vi "Simulate_AirGaps_v1_Core.vi"() -> ()   [LabVIEW 2014]
doc: "I. Description:\nThis example demonstrates how to continuously output a waveform using an internal sample clock. The automatic regeneration of data has been disabled, so new data has to be provided throughout the duration of the continuous Analog Output operation. This allows the generation of any arbitrary frequency as this VI computes new data for each iteration of the loop, maintaining phase continuity of the signal.\n\nII. Instructions for Running:\n1. Select the Physical Channel to correspond to where your signal is output on the DAQ device.\n2. Enter the Minimum and Maximum Voltage range.\n3. Specify the desired Sample Clock Rate of the output Waveform. Higher sample clock rates will produce a smoother waveform.\n4. Manually specify the Analog Output buffer size, in number of samples. A larger buffer would help non-regenerative operations avoid errors due to occasional high CPU load. \nNote: \nThe Analog Output buffer has to be at least as big as the amount of data being written to the board per iteration. The recommended buffer size would be at least twice the amount of data being written to the board per iteration.\n5. Enter the Waveform Information. See the documentation of the Basic Function Generator SubVI for information on each parameter.\n\nIII. Block Diagram Steps:\n1. Create an Analog Output Voltage channel.\n2. Configure the task to prohibit the automatic regeneration of data.\n3. Call the DAQmx (Sample Clock) VI to set the sample clock rate. Additionally, set the sample mode to Continuous.\n4. Read the actual sample clock rate (eventually coerced depending on the hardware used). \n5. Compute the desired waveform, using the buffer size and the actual update rate. This VI keeps track of the phase of the waveform to ensure that the generated signal is continuous.\n6. Write the waveform to the output buffer. \n7a. Call the Start VI. This is only needed when the loop is executed for the first time.\n7b. Do nothing.\n8. Loop continuously until user presses the Stop button. Every iteration computes and writes a new waveform to the buffer.\n9. Call the Clear Task VI to clear the Task.\n10. Use the popup dialog box to display an error or warning if any.\n\nIV. I/O Connections Overview:\nMake sure your signal output terminal matches the Physical Channel I/O Control. For further connection information, refer to your hardware reference manual."
uses:
  <vilib>/Utility/error.llb/DialogType.ctl
  <vilib>/DAQmx/create/channels.llb/DAQmx Create Channel (AO-Voltage-Basic).vi
  <vilib>/DAQmx/configure/timing.llb/DAQmx Timing (Sample Clock).vi
  <vilib>/DAQmx/write.llb/DAQmx Write (Analog 1D Wfm NChan NSamp).vi
  <vilib>/measure/NI_MABase.lvlib
  <resource>/objmgr/daqmx.rc
panel:
  in  "Tab Control":T1(tab)=enum."Air Gap"
  out "Trigger":waveform(dbl)(graph)={"t0"=timestamp(90 s since 1904-01-01), "dt"=0.0005333333333333334, "Y"=array[1500 elements]}
  in  "Trigg. level":sgl=2.0
  in  "Regular level":sgl=10.0
  out "RV":waveform(dbl)[](graph)=[{"t0"=timestamp(90 s since 1904-01-01), "dt"=0.0005333333333333334, "Y"=array[1500 elements]}, {"t0"=timestamp(90 s since 1904-01-01), "dt"=0.0005333333333333334, "Y"=array[1500 elements]}, {"t0"=timestamp(90 s since 1904-01-01), "dt"=0.0005333333333333334, "Y"=array[1500 elements]}, {"t0"=timestamp(90 s since 1904-01-01), "dt"=0.0005333333333333334, "Y"=array[1500 elements]}]
  in  "RV000_Ph":sgl[](array[numeric])=[30.0, 60.0, 90.0]
  in  "RV000_Amp":sgl[](array[numeric])=[1.0, 1.0, 1.0]
  in  "RV000.DC":sgl=5.0
  in  "RV001.DC":sgl=5.0
  in  "RV001_Amp":sgl[](array[numeric])=[1.0, 1.0, 1.0]
  in  "RV001_Ph":sgl[](array[numeric])=[30.0, 60.0, 90.0]
  in  "RV002_Ph":sgl[](array[numeric])=[30.0, 60.0, 90.0]
  in  "RV002_Amp":sgl[](array[numeric])=[1.0, 1.0, 1.0]
  in  "RV002.DC":sgl=5.0
  in  "RV003_Ph":sgl[](array[numeric])=[30.0, 60.0, 90.0]
  in  "RV003_Amp":sgl[](array[numeric])=[1.0, 1.0, 1.0]
  in  "RV003.DC":sgl=5.0
  in  "Multiplication factor":dbl=0.5
  in  "Add Noise":bool
  in  "Change roattion":bool
  in  "First harmonic Phase":sgl=0.1
  out "AG_graph":waveform(dbl)[](graph)
  in  "Pole hight":sgl=6.0
  in  "Add linear increase":bool
  in  "Pole to highlight (from 1 to 72)":i32=166
  in  "Higlight multiplication factor":sgl=1.2
  in  "Offset":sgl=11.0
  in  "increase rate/rotation":sgl=0.5
  in  "Samples to rotate +/100":i32
  in  "First harmonic Amplitude":sgl=0.1
  in  "Add first harmonic":bool
  out "MX":waveform(dbl)(graph)
  in  "MX Amplitude":sgl=1.0
  in  "Pole to highlight (from 1 to 72) MX":i32=166
  in  "Higlight multiplication factor MX":sgl=1.2
  out "Proc1":waveform(dbl)(graph)={"t0"=timestamp(90 s since 1904-01-01), "dt"=0.0005333333333333334, "Y"=array[1500 elements]}
  in  "DC Proc Val 1":sgl=6.0
  out "Proc2":waveform(dbl)(graph)={"t0"=timestamp(90 s since 1904-01-01), "dt"=0.0005333333333333334, "Y"=array[1500 elements]}
  in  "DC Proc Val 2":sgl=6.0
  out "Loop Iteration":dbl=0.7980451583862305
  out "Waveform Graph":waveform(dbl)[](graph)=[{"t0"=timestamp(90 s since 1904-01-01), "dt"=0.0005333333333333334, "Y"=array[1500 elements]}, {"t0"=timestamp(90 s since 1904-01-01), "dt"=0.0005333333333333334, "Y"=array[1500 elements]}, {"t0"=timestamp(90 s since 1904-01-01), "dt"=0.0005333333333333334, "Y"=array[1500 elements]}, {"t0"=timestamp(90 s since 1904-01-01), "dt"=0.0005333333333333334, "Y"=array[1500 elements]}, {"t0"=timestamp(90 s since 1904-01-01), "dt"=0.0005333333333333334, "Y"=array[1500 elements]}, {"t0"=timestamp(90 s since 1904-01-01), "dt"=0.0005333333333333334, "Y"=array[1500 elements]}, {"t0"=timestamp(90 s since 1904-01-01), "dt"=0.0005333333333333334, "Y"=array[1500 elements]}, {"t0"=timestamp(90 s since 1904-01-01), "dt"=0.0005333333333333334, "Y"=array[1500 elements]}, {"t0"=timestamp(90 s since 1904-01-01), "dt"=0.0005333333333333334, "Y"=array[1500 elements]}, {"t0"=timestamp(90 s since 1904-01-01), "dt"=0.0005333333333333334, "Y"=array[1500 elements]}, {"t0"=timestamp(90 s since 1904-01-01), "dt"=0.0005333333333333334, "Y"=array[1500 elements]}] caption="Output Waveforms"
  in  "Physical Channels":tag="Dev2/ao0:11"
  in  "stop":bool
  # "Channel Parameters"
  # "s"
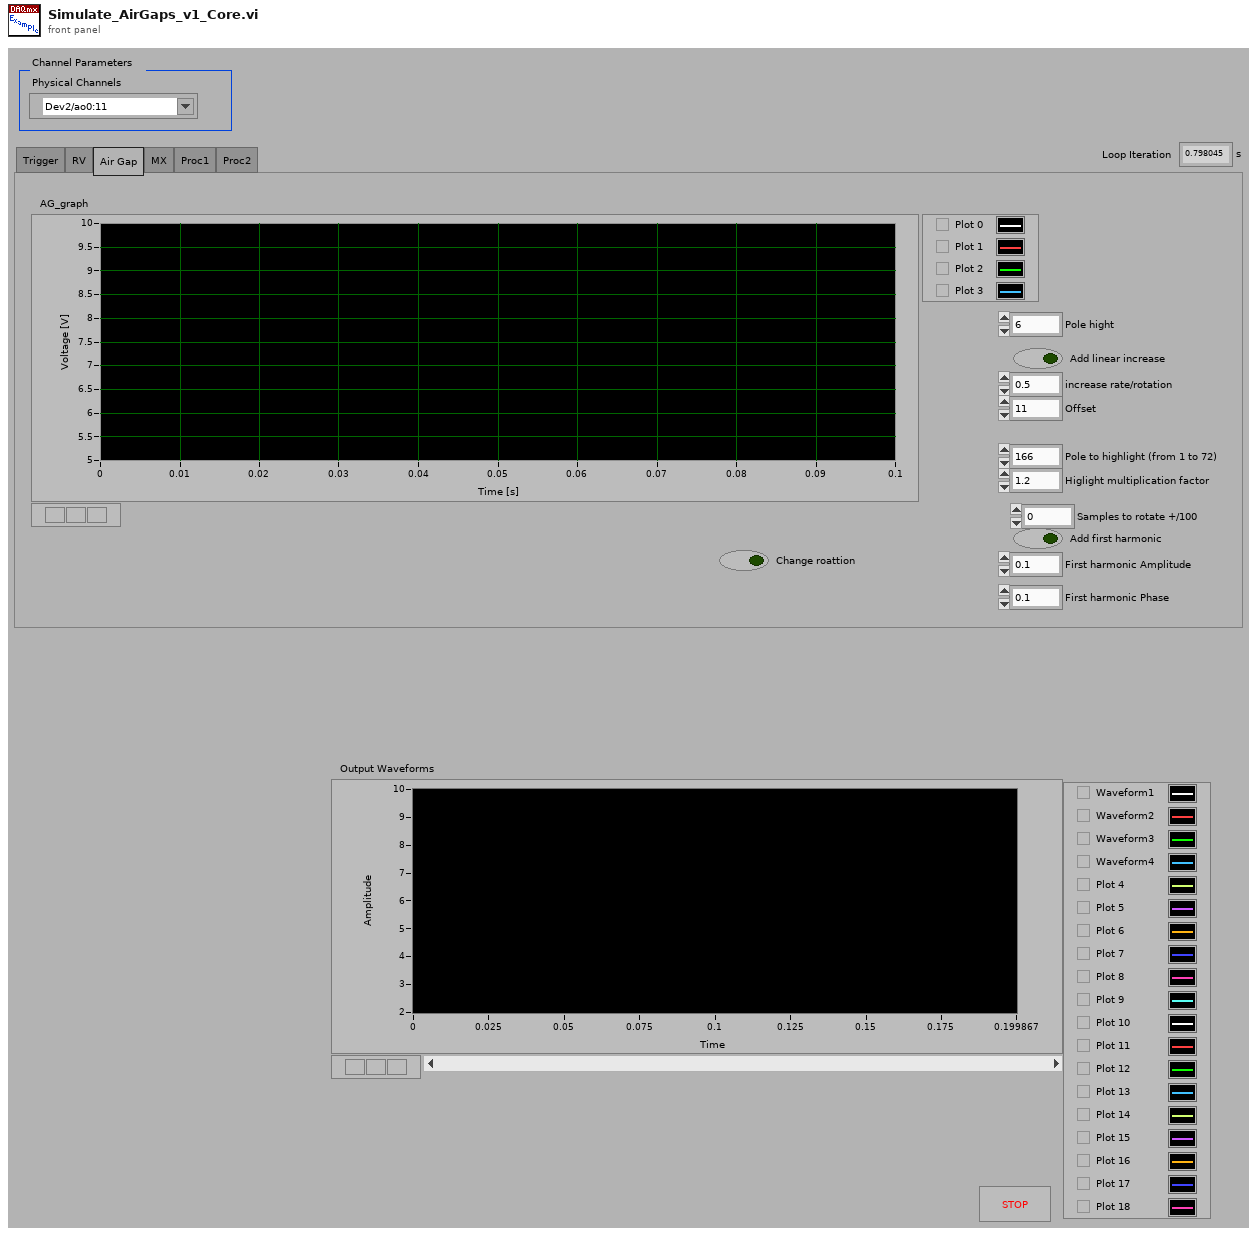
[diagram p1: front panel]
types:
  T1 = enum32{"Trigger", "RV", "Air Gap", "MX", "Proc1", "Proc2"}
  T2 = typedef "DialogType.ctl" = u16
  T3 = enum16{"Sine Wave", "Triangle Wave", "Square Wave", "Sawtooth Wave"}
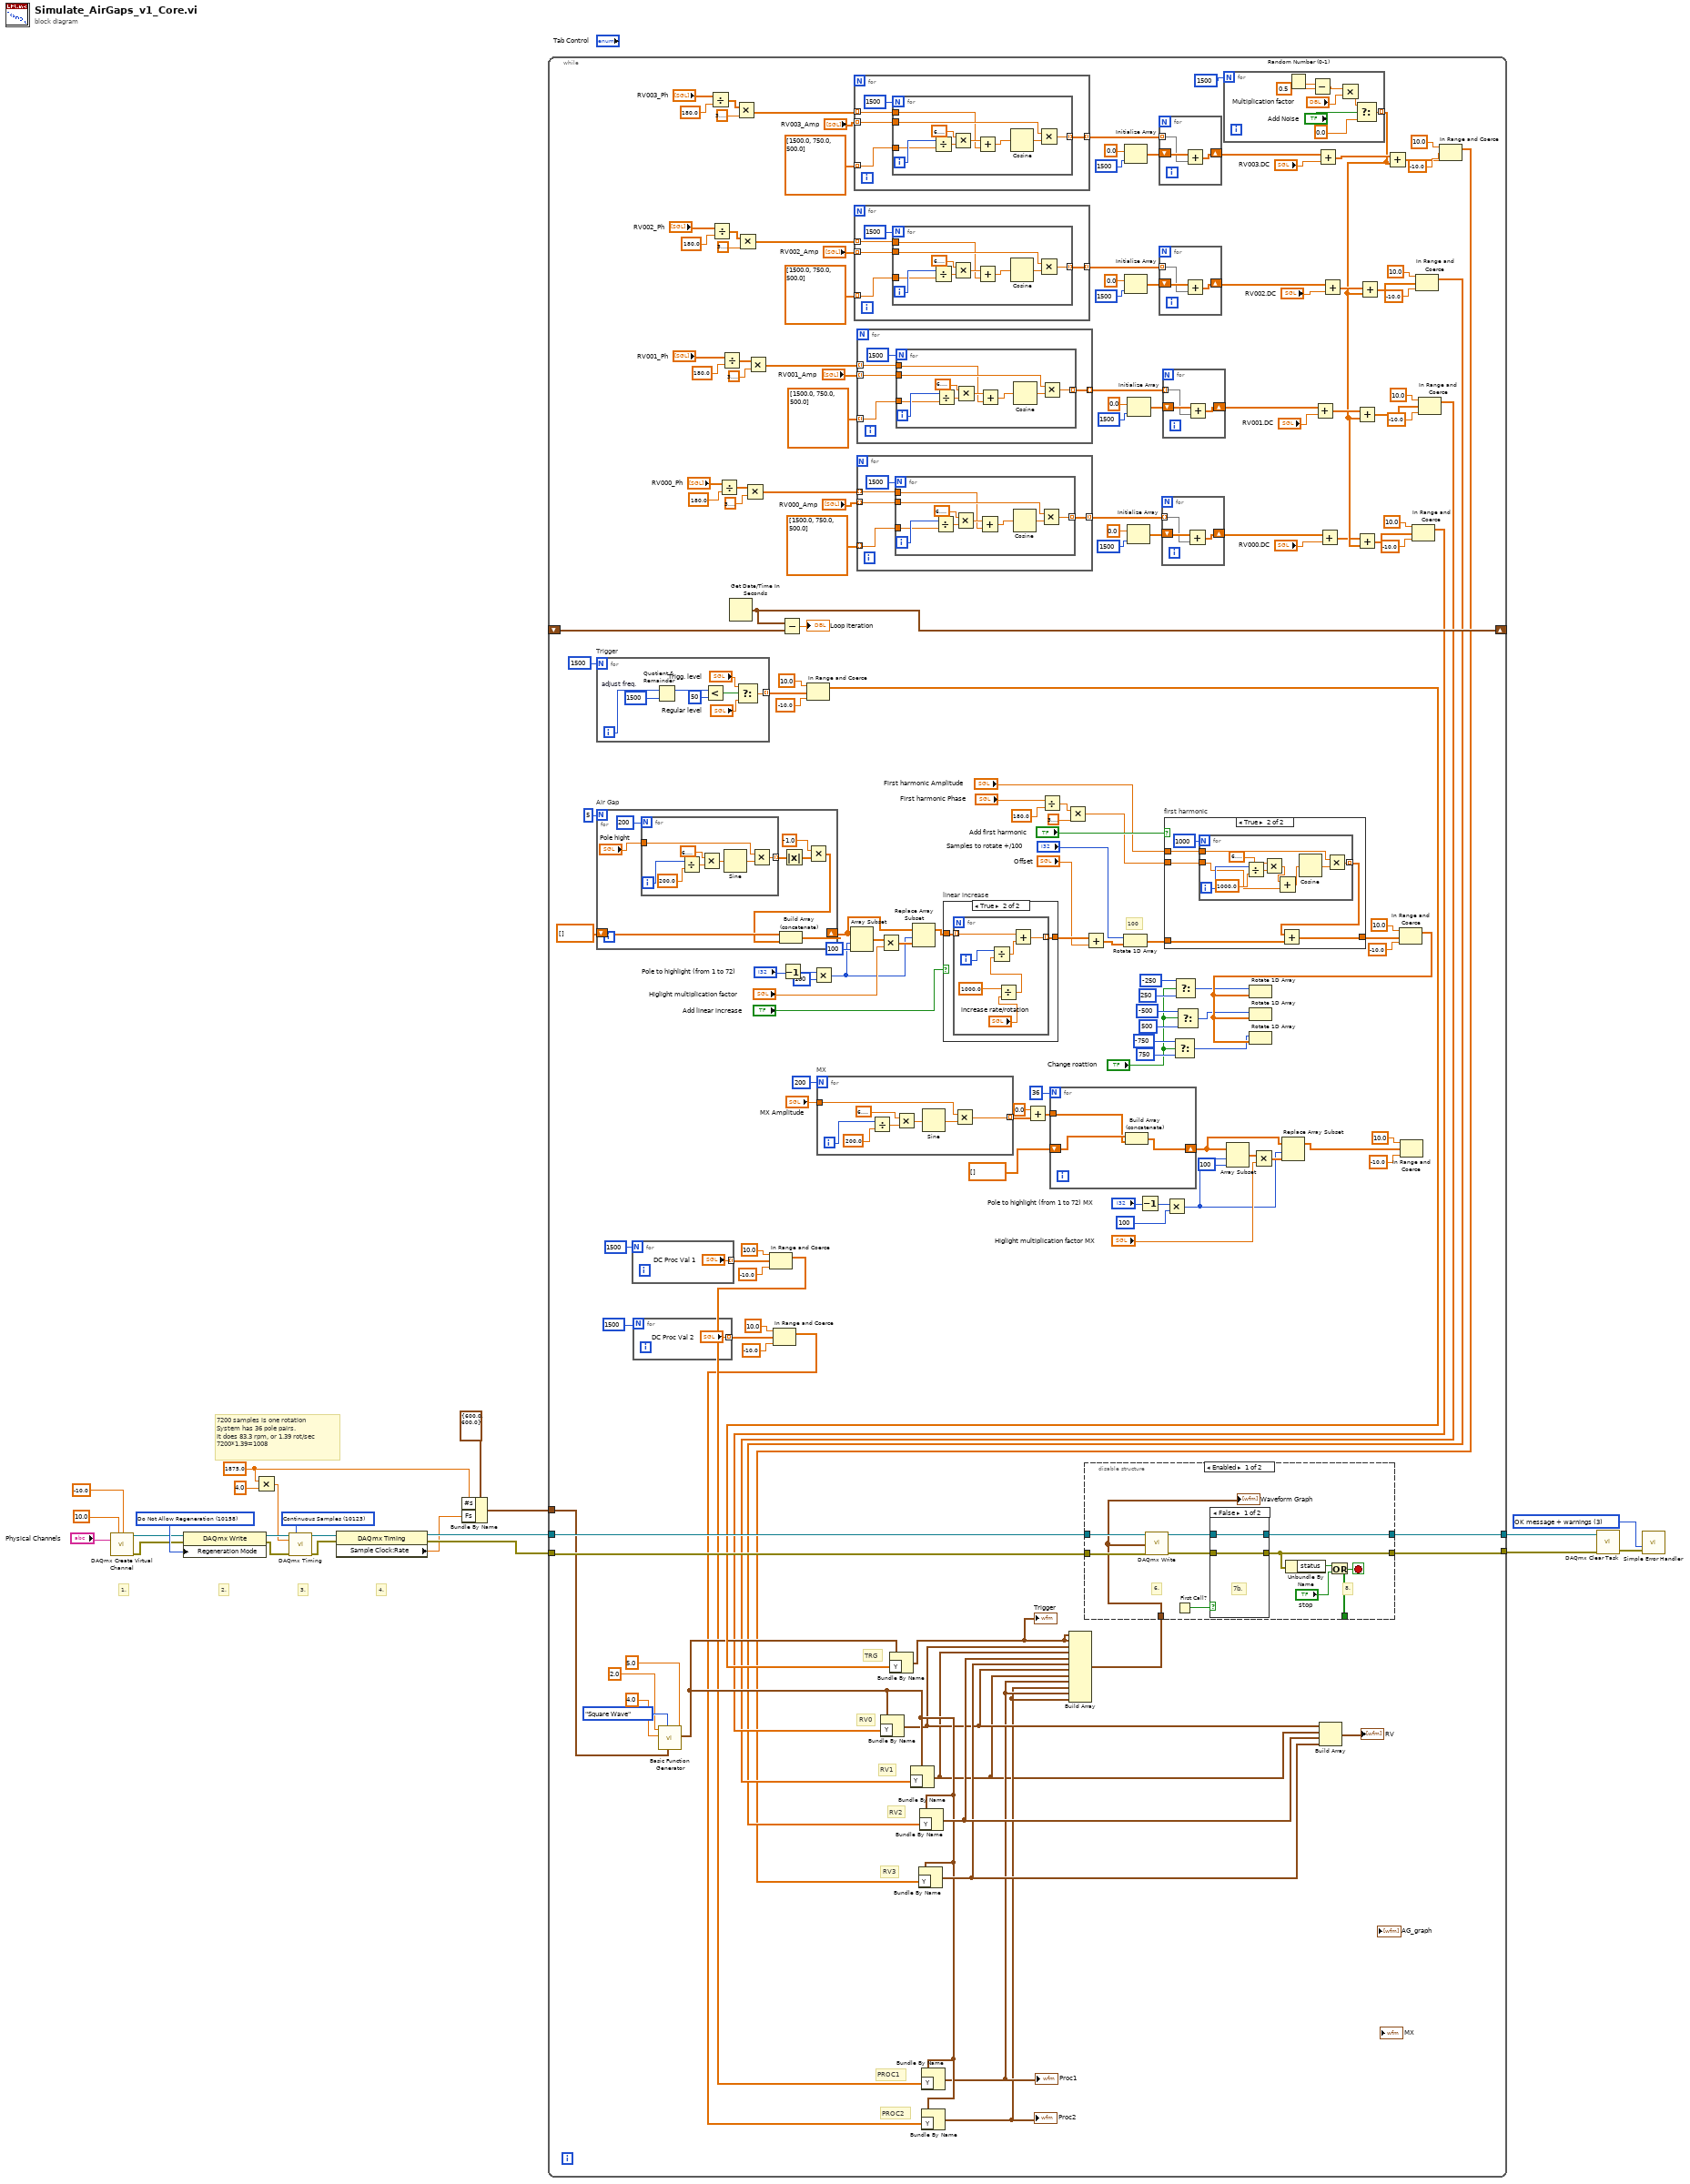
[diagram p0: block diagram]
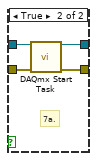
[diagram p2: hidden frame]
diagram:
  w3 = 1875.0 ("Sample Clock Rate")
  w11 = 10158 items=["Allow Regeneration"=10097, "Do Not Allow Regeneration"=10158] ("RegenMode")
  w18 = T2 3 items=["no dialog", "OK message", "continue or stop message", "OK message + warnings", "continue/stop + warnings"] ("type of dialog (OK msg:1)")
  w22 = 10123 items=["Finite Samples"=10178, "Continuous Samples"=10123] ("sample mode")
  # "7200 samples is one rotation\nSystem has 36 pole pairs.\nIt does 83.3 rpm, or 1.39 rot/sec\n7200*1.39=1008"
  # "4."
  # "3."
  # "2."
  # "1."
  n1 = call-poly <vilib>:"DAQmx Create Virtual Channel.vi"("maximum value"=10.0 ("Maximum Value"), "minimum value"=-10.0 ("Minimum Value"), "physical channels"="Physical Channels") -> ("task out"=w10:refnum<k21>, "error out"=w9:errorcluster)  [unwired: 6 in, 5 out]
  n2 = property class="DAQmx Write"(reference=w10, error in=w9, "Regeneration Mode"=w11) -> (reference out=w6:refnum<k21>, error out=w5:errorcluster)
  n3 = Multiply(x=w3, y=4.0) -> (x*y=w1:dbl)
  n4 = call-poly <vilib>:"DAQmx Timing.vi"("task/channels in"=w6, "sample mode"=w22, "rate"=w1, "error in"=w5) -> ("task out"=w15:refnum<k21>, "error out"=w14:errorcluster)  [unwired: 3 in, 7 out]
  n5 = property class="DAQmx Timing"(reference=w15, error in=w14) -> (reference out=w8:refnum<k21>, error out=w7:errorcluster, "Sample Clock:Rate"=w4:dbl)
  n6 = Bundle By Name(cluster=cluster{"Fs":dbl, "#s":dbl} {"Fs"=600.0, "#s"=600.0} ("sampling info"), "#s"=w3, "Fs"=w4) -> (w12:cluster{"Fs":dbl, "#s":dbl})
  n7 = while {
    tunnel: w8 -> [w192]
    tunnel: [w190] -> w17
    tunnel: w7 -> [w189]
    tunnel: [w191] -> w16
    tunnel: w12 -> [w182]
    shift-right: [w188] -> _
    shift-left: _ -> [w177]
    stop <- w193 stop-if-true
    # "PROC2"
    # "PROC1"
    # "RV3"
    # "RV2"
    # "RV1"
    # "TRG"
    # "RV0"
    # "100"
    n8 = for "Trigger" {
      N: 1500 -> [_]
      tunnel: [w348] -> w138 mode=indexing
      i -> [w354]
      w353 = 1500  # adjust freq.
      n9 = Quotient & Remainder(x=w354, y=w353) -> (x-y*floor(x/y)=w352:i32)  [unwired: 1 out]
      n10 = Less?(x=w352, y=50) -> (x < y?=w347:bool)
      n11 = Select(t="Trigg. level", s=w347, f="Regular level") -> (s? t:f=w348:sgl)
    }
    n12 = for "Air Gap" {
      N: 5 -> [_]
      shift-right: [w330] -> w169
      shift-left: sgl[] [] -> [w331]
      n13 = for {
        N: 200 -> [_]
        tunnel: "Pole hight" -> [w338]
        tunnel: [w337] -> w334 mode=indexing
        i -> [w343]
        n14 = Divide(x=w343, y=sgl 200.0) -> (x/y=w342:sgl)
        n15 = Multiply(x=sgl 6.2831855, y=w342) -> (x*y=w340:sgl)
        n16 = Sine(x=w340) -> (sin(x)=w339:sgl)
        n17 = Multiply(x=w338, y=w339) -> (x*y=w337:sgl)
      }
      n18 = Absolute Value(x=w334) -> (abs(x)=w333:sgl[])
      n19 = Multiply(x=sgl -1.0, y=w333) -> (x*y=w329:sgl[])
      n20 = Build Array (concatenate)(w331, w329) -> (w330:sgl[])
    }
    n21 = for {
      N: 1500 -> [_]
      tunnel: ["DC Proc Val 1"] -> w60 mode=indexing
    }
    n22 = for {
      N: 1500 -> [_]
      tunnel: ["DC Proc Val 2"] -> w56 mode=indexing
    }
    n23 = call <vilib>:"Basic Function Generator.vi"("offset"=5.0 ("offset 5"), "sampling info"=w182, "signal type"=T3."Square Wave" ("Waveform Type 5"), "amplitude"=4.0 ("Amplitude 5"), "frequency"=2.0 ("Frequency 5")) -> ("signal out"=w127:waveform(dbl))  [unwired: 4 in, 2 out]
    n24 = Divide(x="RV003_Ph", y=sgl 180.0) -> (x/y=w65:sgl[])
    n25 = Divide(x="RV002_Ph", y=sgl 180.0) -> (x/y=w69:sgl[])
    n26 = Divide(x="RV000_Ph", y=sgl 180.0) -> (x/y=w80:sgl[])
    n27 = Divide(x="RV001_Ph", y=sgl 180.0) -> (x/y=w74:sgl[])
    n28 = Get Date/Time In Seconds() -> (seconds since 1Jan1904=w188:timestamp)
    n29 = Multiply(x=w65, y=sgl 3.1415927) -> (x*y=w63:sgl[])
    n30 = Multiply(x=w69, y=sgl 3.1415927) -> (x*y=w68:sgl[])
    n31 = Multiply(x=w80, y=sgl 3.1415927) -> (x*y=w78:sgl[])
    n32 = Multiply(x=w74, y=sgl 3.1415927) -> (x*y=w73:sgl[])
    n33 = In Range and Coerce(upper limit=sgl 10.0, x=w60, lower limit=sgl -10.0) -> (coerced(x)=w59:sgl[])  [unwired: 1 out]
    n34 = In Range and Coerce(upper limit=sgl 10.0, x=w56, lower limit=sgl -10.0) -> (coerced(x)=w55:sgl[])  [unwired: 1 out]
    n35 = Subtract(x=w188, y=w177) -> (x-y=→"Loop Iteration":dbl)
    n36 = Decrement(x="Pole to highlight (from 1 to 72)") -> (x-1=w167:i32)
    n37 = In Range and Coerce(upper limit=sgl 10.0, x=w138, lower limit=sgl -10.0) -> (coerced(x)=w137:sgl[])  [unwired: 1 out]
    n38 = Multiply(x=w167, y=100) -> (x*y=w165:i32)
    n39 = for "MX" {
      N: 200 -> [_]
      tunnel: "MX Amplitude" -> [w312]
      tunnel: [w311] -> w154 mode=indexing
      i -> [w317]
      n40 = Divide(x=w317, y=sgl 200.0) -> (x/y=w316:sgl)
      n41 = Multiply(x=sgl 6.2831855, y=w316) -> (x*y=w314:sgl)
      n42 = Sine(x=w314) -> (sin(x)=w313:sgl)
      n43 = Multiply(x=w312, y=w313) -> (x*y=w311:sgl)
    }
    n44 = Array Subset(array=w169, index=w165, length=100) -> (w171:sgl[])
    n45 = for {
      tunnel: w63 -> [w225] mode=indexing
      tunnel: "RV003_Amp" -> [w224] mode=indexing
      tunnel: sgl[] [1500.0, 750.0, 500.0] -> [w223] mode=indexing
      tunnel: [w222] -> w99 mode=indexing
      n46 = for {
        N: 1500 -> [_]
        tunnel: w224 -> [w232]
        tunnel: [w231] -> w222 mode=indexing
        tunnel: w225 -> [w228]
        tunnel: w223 -> [w227]
        i -> [w236]
        n47 = Divide(x=w236, y=w227) -> (x/y=w235:sgl)
        n48 = Multiply(x=sgl 6.2831855, y=w235) -> (x*y=w230:sgl)
        n49 = Add(x=w230, y=w228) -> (x+y=w229:sgl)
        n50 = Cosine(x=w229) -> (cos(x)=w233:sgl)
        n51 = Multiply(x=w232, y=w233) -> (x*y=w231:sgl)
      }
    }
    n52 = for {
      tunnel: w68 -> [w243] mode=indexing
      tunnel: "RV002_Amp" -> [w242] mode=indexing
      tunnel: sgl[] [1500.0, 750.0, 500.0] -> [w241] mode=indexing
      tunnel: [w240] -> w102 mode=indexing
      n53 = for {
        N: 1500 -> [_]
        tunnel: w242 -> [w250]
        tunnel: [w249] -> w240 mode=indexing
        tunnel: w243 -> [w246]
        tunnel: w241 -> [w245]
        i -> [w254]
        n54 = Divide(x=w254, y=w245) -> (x/y=w253:sgl)
        n55 = Multiply(x=sgl 6.2831855, y=w253) -> (x*y=w248:sgl)
        n56 = Add(x=w248, y=w246) -> (x+y=w247:sgl)
        n57 = Cosine(x=w247) -> (cos(x)=w251:sgl)
        n58 = Multiply(x=w250, y=w251) -> (x*y=w249:sgl)
      }
    }
    n59 = for {
      tunnel: w78 -> [w279] mode=indexing
      tunnel: "RV000_Amp" -> [w278] mode=indexing
      tunnel: sgl[] [1500.0, 750.0, 500.0] -> [w277] mode=indexing
      tunnel: [w276] -> w126 mode=indexing
      n60 = for {
        N: 1500 -> [_]
        tunnel: w278 -> [w286]
        tunnel: [w285] -> w276 mode=indexing
        tunnel: w279 -> [w282]
        tunnel: w277 -> [w281]
        i -> [w290]
        n61 = Divide(x=w290, y=w281) -> (x/y=w289:sgl)
        n62 = Multiply(x=sgl 6.2831855, y=w289) -> (x*y=w284:sgl)
        n63 = Add(x=w284, y=w282) -> (x+y=w283:sgl)
        n64 = Cosine(x=w283) -> (cos(x)=w287:sgl)
        n65 = Multiply(x=w286, y=w287) -> (x*y=w285:sgl)
      }
    }
    n66 = for {
      tunnel: w73 -> [w261] mode=indexing
      tunnel: "RV001_Amp" -> [w260] mode=indexing
      tunnel: sgl[] [1500.0, 750.0, 500.0] -> [w259] mode=indexing
      tunnel: [w258] -> w117 mode=indexing
      n67 = for {
        N: 1500 -> [_]
        tunnel: w260 -> [w268]
        tunnel: [w267] -> w258 mode=indexing
        tunnel: w261 -> [w264]
        tunnel: w259 -> [w263]
        i -> [w272]
        n68 = Divide(x=w272, y=w263) -> (x/y=w271:sgl)
        n69 = Multiply(x=sgl 6.2831855, y=w271) -> (x*y=w266:sgl)
        n70 = Add(x=w266, y=w264) -> (x+y=w265:sgl)
        n71 = Cosine(x=w265) -> (cos(x)=w269:sgl)
        n72 = Multiply(x=w268, y=w269) -> (x*y=w267:sgl)
      }
    }
    n73 = Multiply(x=w171, y="Higlight multiplication factor") -> (x*y=w168:sgl[])
    n74 = Bundle By Name(cluster=w127, "Y"=w137) -> (w24:waveform(dbl))
    "Trigger" <- w24
    n75 = Replace Array Subset(array=w169, new element=w168, index=w165) -> (w164:sgl[])
    n76 = Bundle By Name(cluster=w127, "Y"=w59) -> (w27:waveform(dbl))
    "Proc1" <- w27
    n77 = Bundle By Name(cluster=w127, "Y"=w55) -> (w26:waveform(dbl))
    "Proc2" <- w26
    n78 = case "linear increase" shown="True" "Add linear increase" {
      tunnel: [w319 w321] -> w161
      tunnel: w164 -> [w319 w320]
      frame False {
      }
      frame True {
        n79 = for {
          tunnel: w320 -> [w328] mode=indexing
          tunnel: [w326] -> w321 mode=indexing
          i -> [w327]
          n80 = Divide(x=sgl 1000.0, y="increase rate/rotation") -> (x/y=w324:sgl)
          n81 = Divide(x=w327, y=w324) -> (x/y=w322:sgl)
          n82 = Add(x=w328, y=w322) -> (x+y=w326:sgl)
        }
      }
    }
    n83 = Add(x=sgl 0.0, y=w154) -> (x+y=w153:sgl[])
    n84 = Divide(x="First harmonic Phase", y=sgl 180.0) -> (x/y=w51:sgl)
    n85 = for {
      N: 36 -> [_]
      tunnel: w153 -> [w308]
      shift-right: [w309] -> w143
      shift-left: sgl[] [] -> [w310]
      n86 = Build Array (concatenate)(w310, w308) -> (w309:sgl[])
    }
    n87 = Multiply(x=w51, y=sgl 3.1415927) -> (x*y=w49:sgl)
    n88 = Add(x=w161, y="Offset") -> (x+y=w134:sgl[])
    n89 = Rotate 1D Array(1:w134, 2:"Samples to rotate +/100") -> (0:w136:sgl[])
    n90 = Initialize Array(sgl 0.0, 1500 ("dimension size")) -> (w95:sgl[])
    n91 = Initialize Array(sgl 0.0, 1500 ("dimension size")) -> (w106:sgl[])
    n92 = Initialize Array(sgl 0.0, 1500 ("dimension size")) -> (w121:sgl[])
    n93 = Initialize Array(sgl 0.0, 1500 ("dimension size")) -> (w113:sgl[])
    n94 = Decrement(x="Pole to highlight (from 1 to 72) MX") -> (x-1=w149:i32)
    n95 = for {
      shift-right: [w219] -> w84
      shift-left: w95 -> [w221]
      tunnel: w99 -> [w220] mode=indexing
      n96 = Add(x=w221, y=w220) -> (x+y=w219:sgl[])
    }
    n97 = for {
      shift-right: [w237] -> w86
      shift-left: w106 -> [w239]
      tunnel: w102 -> [w238] mode=indexing
      n98 = Add(x=w239, y=w238) -> (x+y=w237:sgl[])
    }
    n99 = for {
      shift-right: [w273] -> w90
      shift-left: w121 -> [w275]
      tunnel: w126 -> [w274] mode=indexing
      n100 = Add(x=w275, y=w274) -> (x+y=w273:sgl[])
    }
    n101 = for {
      shift-right: [w255] -> w88
      shift-left: w113 -> [w257]
      tunnel: w117 -> [w256] mode=indexing
      n102 = Add(x=w257, y=w256) -> (x+y=w255:sgl[])
    }
    n103 = case "first harmonic" shown="True" "Add first harmonic" {
      tunnel: w136 -> [w291 w296]
      tunnel: [w291 w294] -> w133
      tunnel: "First harmonic Amplitude" -> [_ w293]
      tunnel: w49 -> [_ w292]
      frame False {
      }
      frame True {
        n104 = for {
          N: 1000 -> [_]
          tunnel: w293 -> [w302]
          tunnel: [w301] -> w295 mode=indexing
          tunnel: w292 -> [w299]
          i -> [w306]
          n105 = Divide(x=w306, y=sgl 1000.0) -> (x/y=w305:sgl)
          n106 = Multiply(x=sgl 6.2831855, y=w305) -> (x*y=w300:sgl)
          n107 = Add(x=w300, y=w299) -> (x+y=w298:sgl)
          n108 = Cosine(x=w298) -> (cos(x)=w303:sgl)
          n109 = Multiply(x=w302, y=w303) -> (x*y=w301:sgl)
        }
        n110 = Add(x=w295, y=w296) -> (x+y=w294:sgl[])
      }
    }
    n111 = Multiply(x=w149, y=100) -> (x*y=w144:i32)
    n112 = Select(t=-750 ("n"), s="Change roattion", f=750 ("n")) -> (s? t:f=w30:i32)
    n113 = Select(t=-250 ("n"), s="Change roattion", f=250 ("n")) -> (s? t:f=w32:i32)
    n114 = Select(t=-500 ("n"), s="Change roattion", f=500 ("n")) -> (s? t:f=w31:i32)
    n115 = for {
      N: 1500 -> [_]
      tunnel: [w211] -> w41 mode=indexing
      n116 = Random Number (0-1)() -> (number: 0 to 1=w216:dbl)
      n117 = Subtract(x=w216, y=0.5) -> (x-y=w214:dbl)
      n118 = Multiply(x=w214, y="Multiplication factor") -> (x*y=w212:dbl)
      n119 = Select(t=w212, s="Add Noise", f=0.0) -> (s? t:f=w211:dbl)
    }
    n120 = Array Subset(array=w143, index=w144, length=100) -> (w147:sgl[])
    n121 = Multiply(x=w147, y="Higlight multiplication factor MX") -> (x*y=w145:sgl[])
    n122 = Replace Array Subset(array=w143, new element=w145, index=w144) -> (w132:sgl[])
    n123 = Add(x=w88, y="RV001.DC") -> (x+y=w43:sgl[])
    n124 = Add(x=w84, y="RV003.DC") -> (x+y=w47:sgl[])
    n125 = Add(x=w90, y="RV000.DC") -> (x+y=w40:sgl[])
    n126 = Add(x=w86, y="RV002.DC") -> (x+y=w45:sgl[])
    n127 = Add(x=w43, y=w41) -> (x+y=w42:dbl[])
    n128 = Add(x=w40, y=w41) -> (x+y=w39:dbl[])
    n129 = Add(x=w45, y=w41) -> (x+y=w44:dbl[])
    n130 = Add(x=w47, y=w41) -> (x+y=w46:dbl[])
    n131 = In Range and Coerce(upper limit=sgl 10.0, x=w133, lower limit=sgl -10.0) -> (coerced(x)=w128:sgl[])  [unwired: 1 out]
    n132 = Rotate 1D Array(1:w128, 2:w32) -> ()  [unwired: 1 out]
    n133 = Rotate 1D Array(1:w128, 2:w31) -> ()  [unwired: 1 out]
    n134 = Rotate 1D Array(1:w128, 2:w30) -> ()  [unwired: 1 out]
    n135 = In Range and Coerce(upper limit=sgl 10.0, x=w132, lower limit=sgl -10.0) -> ()  [unwired: 2 out]
    n136 = In Range and Coerce(upper limit=sgl 10.0, x=w39, lower limit=sgl -10.0) -> (coerced(x)=w118:dbl[])  [unwired: 1 out]
    n137 = Bundle By Name(cluster=w127, "Y"=w118) -> (w28:waveform(dbl))
    n138 = In Range and Coerce(upper limit=sgl 10.0, x=w44, lower limit=sgl -10.0) -> (coerced(x)=w100:dbl[])  [unwired: 1 out]
    n139 = Bundle By Name(cluster=w127, "Y"=w100) -> (w131:waveform(dbl))
    n140 = In Range and Coerce(upper limit=sgl 10.0, x=w42, lower limit=sgl -10.0) -> (coerced(x)=w109:dbl[])  [unwired: 1 out]
    n141 = Bundle By Name(cluster=w127, "Y"=w109) -> (w25:waveform(dbl))
    n142 = In Range and Coerce(upper limit=sgl 10.0, x=w46, lower limit=sgl -10.0) -> (coerced(x)=w91:dbl[])  [unwired: 1 out]
    n143 = Bundle By Name(cluster=w127, "Y"=w91) -> (w130:waveform(dbl))
    n144 = Build Array(w24, w24, w28, w25, w131, w130, w28, w25, w27, w26, w27, w26) -> (w181:waveform(dbl)[])
    n145 = disable-structure shown="Enabled" {
      disable-tunnel: [w204 _] -> w193
      disable-tunnel: w192 -> [w201 _]
      disable-tunnel: [w198 _] -> w191
      disable-tunnel: [w197 _] -> w190
      disable-tunnel: w189 -> [w195 _]
      disable-tunnel: w181 -> [w194 _]
      frame Enabled {
        # "8."
        # "6."
        n146 = call-poly <vilib>:"DAQmx Write.vi"("task/channels in"=w201, "data"=w194, "error in"=w195) -> ("task out"=w200:refnum<k21>, "error out"=w199:errorcluster)  [unwired: 1 in, 10 out]
        n147 = First Call?() -> (First Call?: T/F=w196:bool)
        n148 = case shown="False" w196 {
          tunnel: w200 -> [w206 w210]
          tunnel: w199 -> [w205 w209]
          tunnel: [w205 w208] -> w198
          tunnel: [w206 w207] -> w197
          frame False {
            # "7b."
          }
          frame True {
            # "7a."
            n149 = call <vilib>:"DAQmx Start Task.vi"("task/channels in"=w210, "error in"=w209) -> ("task out"=w207:refnum<k21>, "error out"=w208:errorcluster)  [unwired: 12 out]
          }
        }
        n150 = Unbundle By Name(w198) -> ("status"=w203:bool)
        n151 = Or(x=w203, y="stop") -> (x .or. y?=w204:bool)
        "Waveform Graph" <- w194
      }
      frame Disabled {
      }
    }
    n152 = Build Array(w28, w25, w131, w130) -> (→"RV":waveform(dbl)[])
  }
  n153 = call <vilib>:"DAQmx Clear Task.vi"("task in"=w17, "error in"=w16) -> ("error out"=w23:errorcluster)  [unwired: 13 out]
  n154 = call <vilib>:"Simple Error Handler.vi"("type of dialog (OK msg:1)"=w18, "error in (no error)"=w23) -> ()  [unwired: 8 out]
